vi "Create CPU Info.vi"(8 "error in (no error)":errorcluster) -> (0 "error out":errorcluster, 3 "CPU Info out":refnum<class "CPU Info.lvclass">)   [LabVIEW 2019, in "DSF Core.lvlib" / "CPU Info.lvclass"]
uses:
  CPU Info.lvclass
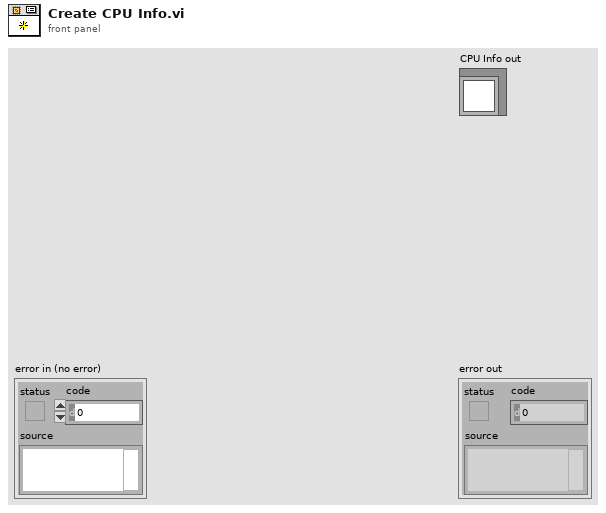
[diagram p1: front panel]
types:
  T1 = cluster{"total cache size":i32, "cache entry size":i32}[]
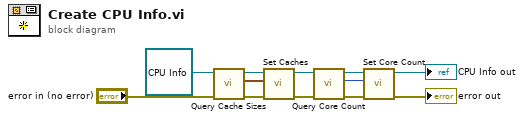
[diagram p0: block diagram]
diagram:
  n1 = call "Query Cache Sizes.vi"("error in (no error)"="error in (no error)", "CPU Info in"=refnum<class "CPU Info.lvclass"> refnum) -> ("error out"=w9:errorcluster, "Caches"=w8:T1, "CPU Info out"=w10:refnum<class "CPU Info.lvclass">)  [unwired: 7 in]
  n2 = call "Set Caches.vi"("error in (no error)"=w9, "Caches"=w8, "CPU Info in"=w10) -> ("error out"=w6:errorcluster, "CPU Info out"=w7:refnum<class "CPU Info.lvclass">)  [unwired: 7 in]
  n3 = call "Query Core Count.vi"("error in (no error)"=w6, "CPU Info in"=w7) -> ("error out"=w4:errorcluster, "Core Count"=w3:i32, "CPU Info out"=w5:refnum<class "CPU Info.lvclass">)  [unwired: 7 in]
  n4 = call "Set Core Count.vi"("error in (no error)"=w4, "Core Count"=w3, "CPU Info in"=w5) -> ("error out"=→"error out":errorcluster, "CPU Info out"=→"CPU Info out":refnum<class "CPU Info.lvclass">)  [unwired: 7 in]
